vi "test.vi"() -> ()   [LabVIEW 2010]
panel:
  out "Balance 2":i32
  in  "Balance":dbl(slide) scale=1000.0..-1000.0
  out "ErrorDescription":string
  out "ErrorCode":i32
  out "ReadyState":i32(ring) items=["mpReadyStateUninitialized"=0, "mpReadyStateLoading"=1, "mpReadyStateInteractive"=3, "mpReadyStateComplete"=4]
  in  "mute":bool
  in  "Position":ext(slide) scale=-1.0..292.83825
  in  "Pfad":path=path "D:/Musik/Geld oder Leben/Einsamkeit.mp3"
  in  "stop":bool
  out "error_pool":errorcluster caption="Fehler (Ausgang)"
  out "PlayState":i32(ring) items=["mpStopped", "mpPaused", "mpPlaying", "mpWaiting", "mpScanForward", "mpScanReverse", "mpClosed"]
  out "aktuell":string="00 : 00 :  0"
  out "Zeit insgsamt":string="00 : 00 :  0"
  out "Duration":i32 format="%.2f"
  in  "Volume":dbl(slide)
  out "Fehler (Ausgang)":errorcluster
  in  "pause":bool
  in  "stoppen":bool
  in  "play":bool
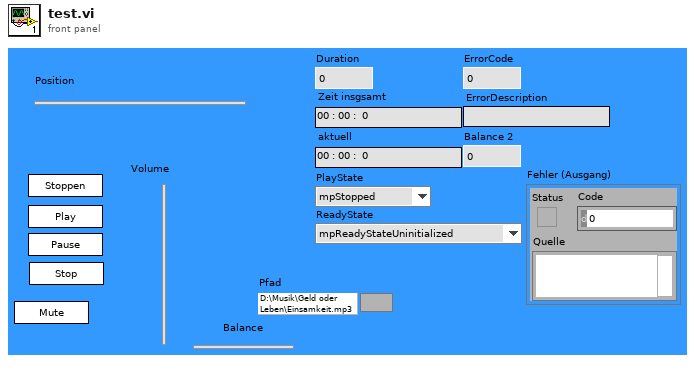
[diagram p1: front panel]
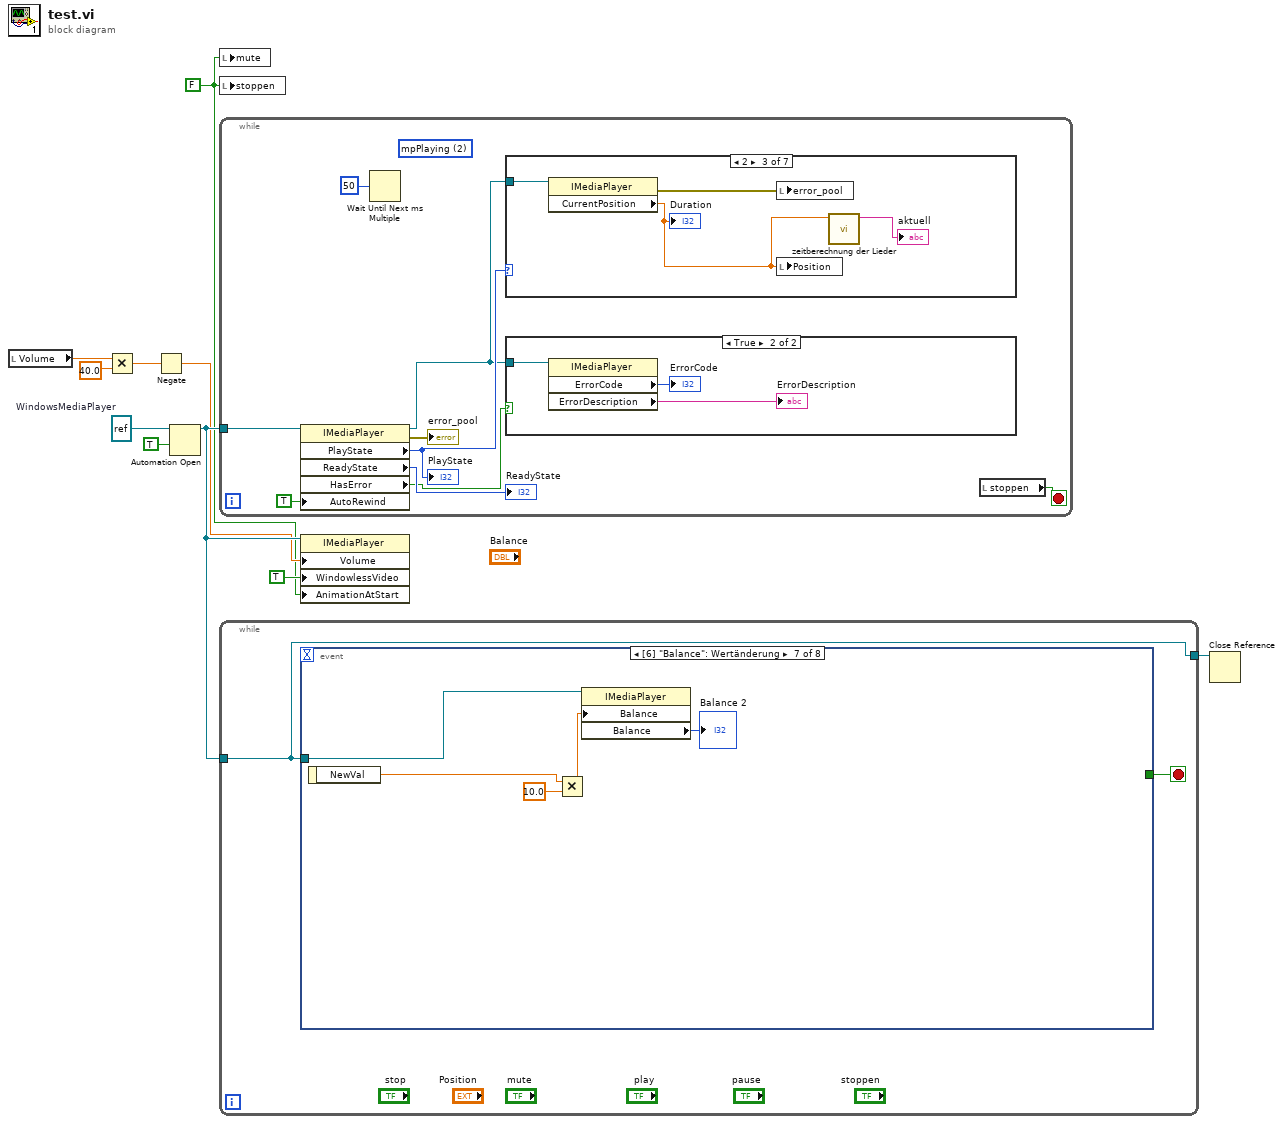
[diagram p0: block diagram]
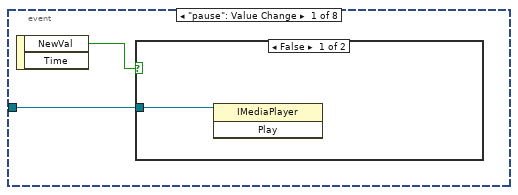
[diagram p9: hidden frame]
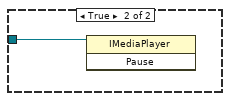
[diagram p10: hidden frame]
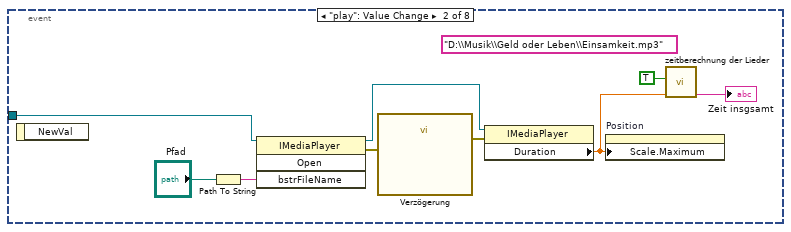
[diagram p11: hidden frame]
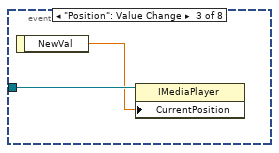
[diagram p12: hidden frame]
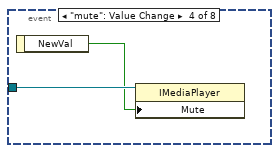
[diagram p13: hidden frame]
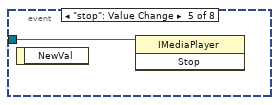
[diagram p14: hidden frame]
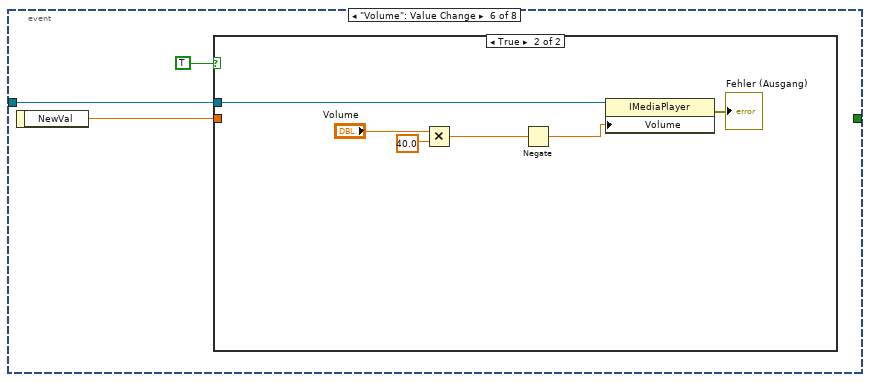
[diagram p15: hidden frame]
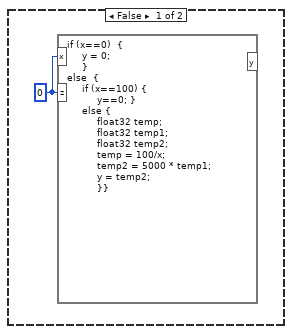
[diagram p16: hidden frame]
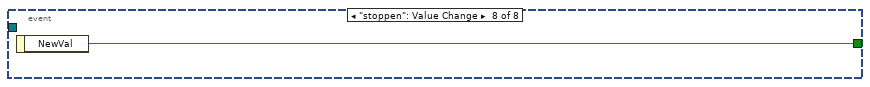
[diagram p17: hidden frame]
diagram:
  w1 = FALSE ("stop")
  w10 = refnum<k7> refnum  # WindowsMediaPlayer
  n1 = local read "Volume"() -> (w3:dbl)
  n2 = Multiply(x=w3, y=40.0) -> (x*y=w6:dbl)
  n3 = Negate(x=w6) -> (-x=w4:dbl)
  n4 = Automation Open(Automation Refnum=w10, 9:TRUE ("Neue Instanz öffnen (False)")) -> (Automation Refnum=w7:refnum<k7>)  [unwired: 2 in, 1 out]
  n5 = local write "mute"(w1) -> ()
  n6 = local write "stoppen"(w1) -> ()
  n7 = while {
    tunnel: w7 -> [w17]
    stop <- w18 stop-if-true
    (unwired) 2 items=["mpStopped", "mpPaused", "mpPlaying", "mpWaiting", "mpScanForward", "mpScanReverse", "mpClosed"] ("PlayState")
    n8 = property class="IMediaPlayer"(reference=w17, "AutoRewind"=TRUE) -> (reference out=w12:refnum<k7>, error out=→"error_pool":errorcluster, "PlayState"=w16:i32, "ReadyState"=→"ReadyState":i32, "HasError"=w13:bool)  [unwired: 1 in]
    "PlayState" <- w16
    n9 = Wait Until Next ms Multiple(millisecond multiple=u32 50 ("Vielfache von ms")) -> ()  [unwired: 1 out]
    n10 = case shown="2" w16 {
      tunnel: w12 -> [_ _ w25 _ _ _ _]
      frame 0, Default {
      }
      frame 1 {
      }
      frame 2 {
        n11 = property class="IMediaPlayer"(reference=w25) -> (error out=w24:errorcluster, "CurrentPosition"=w23:dbl)  [unwired: 1 in, 1 out]
        "Duration" <- w23
        n12 = local write "error_pool"(w24) -> ()
        n13 = local write "Position"(w23) -> ()
        n14 = call "zeitberechnung der Lieder.vi"("aktuell"=w23) -> ("aktuell"=→"aktuell":string)  [unwired: 9 in, 1 out]
      }
      frame 3 {
      }
      frame 4 {
      }
      frame 5 {
      }
      frame 6 {
      }
    }
    n15 = case shown="True" w13 {
      tunnel: w12 -> [_ w22]
      frame False {
      }
      frame True {
        n16 = property class="IMediaPlayer"(reference=w22) -> ("ErrorCode"=→"ErrorCode":i32, "ErrorDescription"=→"ErrorDescription":string)  [unwired: 1 in, 2 out]
      }
    }
    n17 = local read "stoppen"() -> (w18:bool)
  }
  n18 = while {
    tunnel: w7 -> [w28]
    tunnel: [w28] -> w8
    stop <- w27 stop-if-true
    n19 = event shown="[6] \"Balance\": Wertänderung" {
      selector: _ -> [_ _ _ _ _ _ _ _]
      dyn-events: _ -> [_ _ _ _ _ _ _ _]
      timeout: _ -> [_ _ _ _ _ _ _ _]
      tunnel: w28 -> [w29 w41 w43 w45 w46 w49 w58 _]
      tunnel: [_ _ _ _ _ _ _ w62] -> w27
      event "pause": Value Change {
        n20 = event-data() -> ("NewVal"=w30:bool)  [unwired: 1 in, 1 out]
        n21 = case shown="False" w30 {
          tunnel: w29 -> [w31 w32]
          frame False {
            n22 = invoke class="IMediaPlayer" method="Play"(reference=w31) -> ()  [unwired: 2 in, 3 out]
          }
          frame True {
            n23 = invoke class="IMediaPlayer" method="Pause"(reference=w32) -> ()  [unwired: 2 in, 3 out]
          }
        }
      }
      event "play": Value Change {
        (unwired) "D:\\Musik\\Geld oder Leben\\Einsamkeit.mp3" ("BaseURL")
        n24 = event-data() -> ()  [unwired: 1 in, 1 out]
        n25 = Path To String(path="Pfad") -> (string=w34:string)
        n26 = invoke class="IMediaPlayer" method="Open"(reference=w41, "bstrFileName"=w34) -> (reference out=w40:refnum<k7>, error out=w37:errorcluster)  [unwired: 2 in, 2 out]
        n27 = call "Verzögerung"("error in (no error)"=w37) -> ("error out"=w36:errorcluster)  [unwired: 10 in]
        n28 = property class="IMediaPlayer"(reference=w40, error in=w36) -> ("Duration"=w33:dbl)  [unwired: 2 out]
        n29 = property on="Position" class="Schieber (strikt)"("Scale.Maximum"=w33) -> ()  [unwired: 2 in, 2 out]
        n30 = call "zeitberechnung der Lieder.vi"("Zeit insgesamt"=w33, "insgesamt?"=TRUE) -> ("Zeit insgsamt"=→"Zeit insgsamt":string)  [unwired: 8 in, 1 out]
      }
      event "Position": Value Change {
        n31 = event-data() -> ("NewVal"=w42:ext)  [unwired: 1 in]
        n32 = property class="IMediaPlayer"(reference=w43, "CurrentPosition"=w42) -> ()  [unwired: 1 in, 2 out]
      }
      event "mute": Value Change {
        n33 = event-data() -> ("NewVal"=w44:bool)  [unwired: 1 in]
        n34 = property class="IMediaPlayer"(reference=w45, "Mute"=w44) -> ()  [unwired: 1 in, 2 out]
      }
      event "stop": Value Change {
        n35 = event-data() -> ()  [unwired: 1 in, 1 out]
        n36 = invoke class="IMediaPlayer" method="Stop"(reference=w46) -> ()  [unwired: 2 in, 3 out]
      }
      event "Volume": Value Change {
        n37 = event-data() -> ("NewVal"=w48:dbl)  [unwired: 1 in]
        n38 = case shown="True" TRUE {
          tunnel: w49 -> [_ w56]
          tunnel: w48 -> [_ _]
          frame False {
            w50 = 0
            n39 = formula code="if (x==0)  {\n     y = 0; \n     }\nelse  {\n     if (x==100) {\n          y==0; }\n     else {\n          float32 temp;\n          float32 temp1;\n          float32 temp2;\n          temp = 100/x;\n          temp2 = 5000 * temp1;\n          y = temp2;\n          }}"("x"=w50, "z"=w50) -> ()  [unwired: 1 out]
          }
          frame True {
            n40 = Multiply(x="Volume", y=40.0) -> (x*y=w53:dbl)
            n41 = Negate(x=w53) -> (-x=w51:dbl)
            n42 = property class="IMediaPlayer"(reference=w56, "Volume"=w51) -> (error out=→"Fehler (Ausgang)":errorcluster)  [unwired: 1 in, 1 out]
          }
        }
      }
      event "Balance": Value Change {
        n43 = event-data() -> ("NewVal"=w61:dbl)  [unwired: 1 in]
        n44 = Multiply(x=w61, y=10.0) -> (x*y=w59:dbl)
        n45 = property class="IMediaPlayer"(reference=w58, "Balance"=w59) -> ("Balance"=→"Balance 2":i32)  [unwired: 1 in, 2 out]
      }
      event "stoppen": Value Change {
        n46 = event-data() -> ("NewVal"=w62:bool)  [unwired: 1 in]
      }
    }
  }
  n47 = property class="IMediaPlayer"(reference=w7, "Volume"=w4, "WindowlessVideo"=TRUE ("Enabled"), "AnimationAtStart"=w1) -> ()  [unwired: 1 in, 2 out]
  n48 = Close Reference(reference=w8) -> ()  [unwired: 1 in, 1 out]
